vi "knob2.vi"(2 "error in (no error)":errorcluster) -> (0 "error out":errorcluster, 1 "Within Limit 2":bool=TRUE, 3 "Value":dbl)   [LabVIEW 2021]
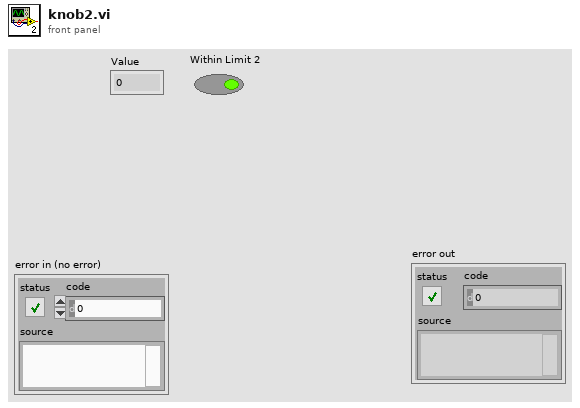
[diagram p1: front panel]
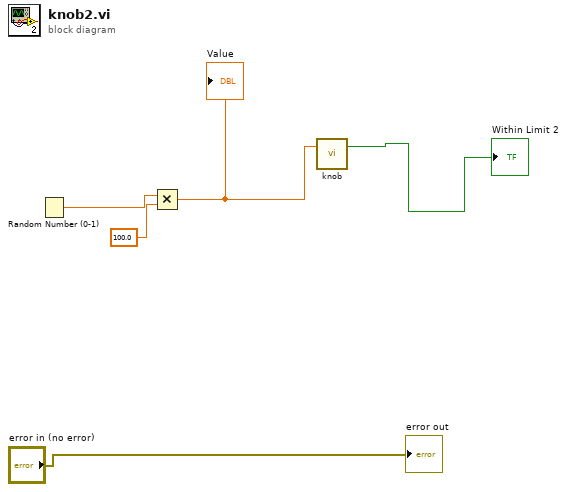
[diagram p0: block diagram]
diagram:
  n1 = Random Number (0-1)() -> (number: 0 to 1=w3:dbl)
  n2 = Multiply(x=w3, y=100.0) -> (x*y=w1:dbl)
  "Value" <- w1
  n3 = call "knob.vi"("Value"=w1) -> ("Within Limit"=→"Within Limit 2":bool)  [unwired: 1 in, 1 out]
  "error out" <- "error in (no error)"
